vi "mod_GSM Integrate Bits.vi"(0 "bit burst in":i8[](array[numeric]), 1 "reference index":i32, 2 "reference value":i8) -> (3 "GSM integrated bit burst":i8[](array[numeric]))   [LabVIEW 2020, in "niDMT.lvlib"]
uses:
  <vilib>/addons/Modulation/niDMT.lvlib
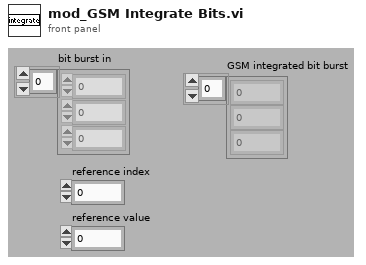
[diagram p1: front panel]
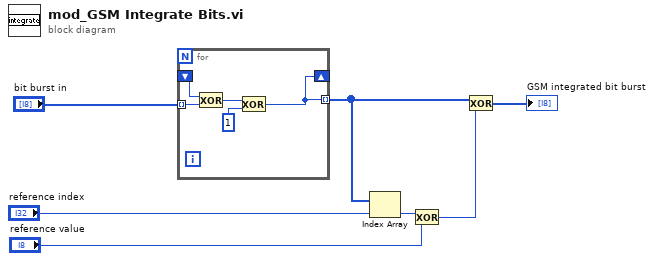
[diagram p0: block diagram]
diagram:
  n1 = for {
    tunnel: "bit burst in" -> [w11] mode=indexing
    tunnel: [w8] -> w7 mode=indexing
    shift-right: [w8] -> _
    shift-left: _ -> [w12]
    n2 = Exclusive Or(1:w11, 2:w12) -> (0:w10:i8)
    n3 = Exclusive Or(1:i8 1 ("y"), 2:w10) -> (0:w8:i8)
  }
  n4 = Index Array(array=w7, index="reference index") -> (element=w5:i8)
  n5 = Exclusive Or(1:"reference value", 2:w5) -> (0:w2:i8)
  n6 = Exclusive Or(1:w2, 2:w7) -> (0:→"GSM integrated bit burst":i8[])
